vi "check asynchronous errors.vi"(8 "error in":errorcluster, 11 "Module Info In":T1) -> (0 "error out":errorcluster, 2 "safe state?":bool, 3 "Module Info Out":T1)   [LabVIEW 2013, in "Standard Engine Runtime.lvclass"]
uses:
  Standard Engine Runtime.lvclass
  async execution info.ctl
  asynchronous process data.ctl
  async command notification.ctl
  <vilib>/NI/Tag Bus/table/data table.ctl
  <vilib>/NI/Tag Bus Module Framework/runtime/execution settings.ctl
  async error info.ctl
  <vilib>/NI/Tag Bus Module Framework/runtime/error classification.ctl
  Data Table with Transfer Spec.ctl
  <vilib>/NI/Tag Bus/table/transfer specification.ctl
  <vilib>/NI/Tag Bus/tag/Data Type.ctl
  Configuration/Module Decimation.ctl
  Configuration/Module Error Configuration.ctl
  Configuration/Error Actions By Category.ctl
  Configuration/Error Actions.ctl
  Configuration/Standard Engine Configuration.lvclass
  <vilib>/NI/Tag Bus Module Framework/runtime/TBM module execution interface.lvclass
  <vilib>/NI/Tag Bus/tag/tag descriptor.lvclass
  <vilib>/NI/Tag Bus/table/data table.lvlib
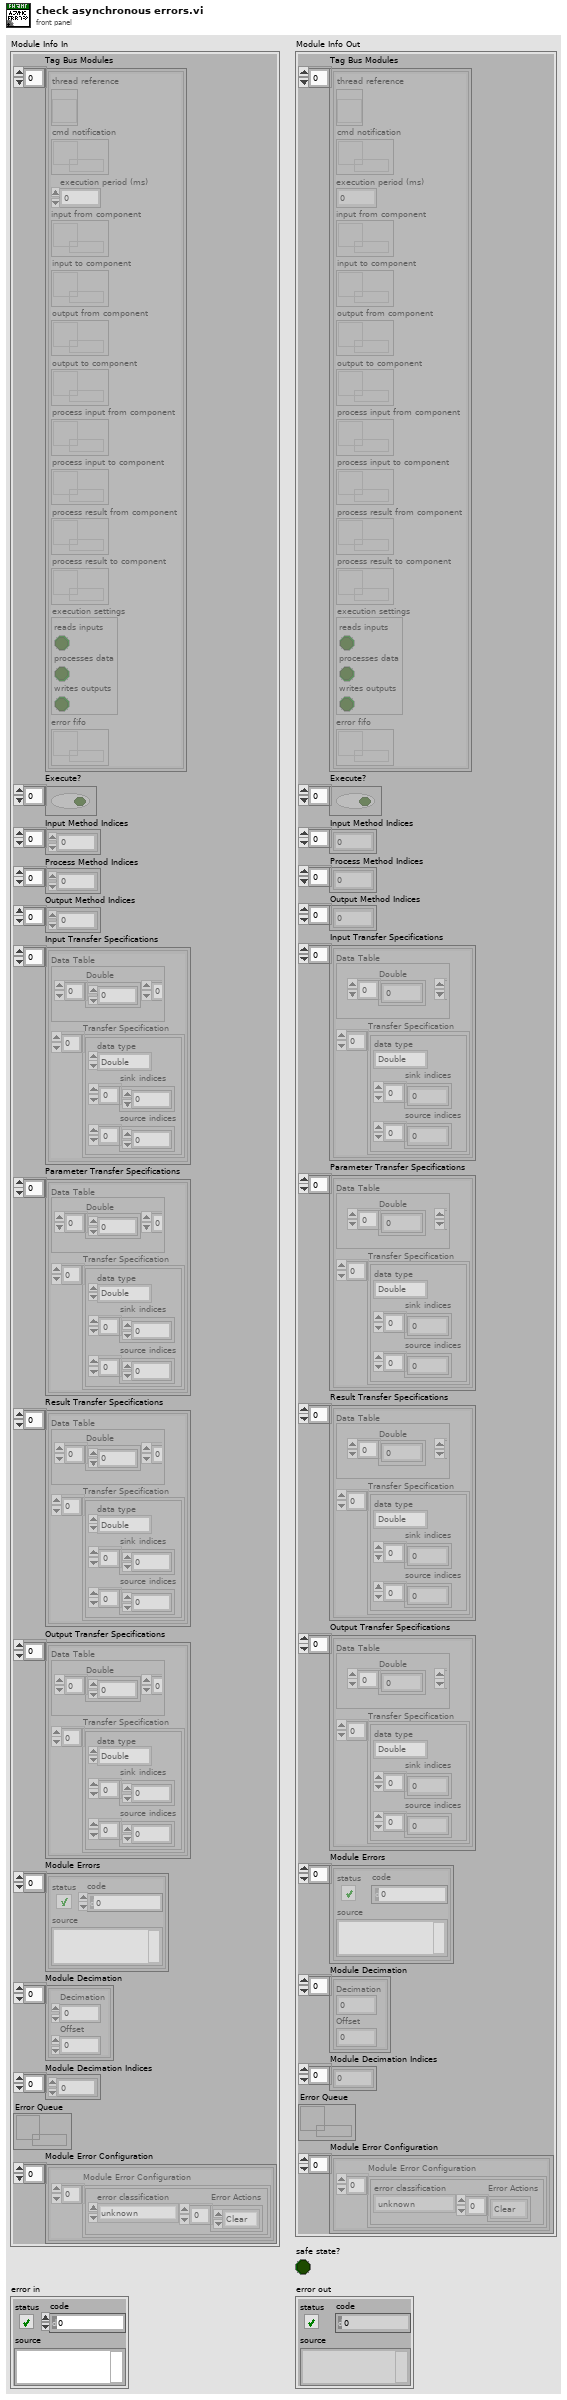
[diagram p1: front panel]
types:
  T1 = typedef "Standard Engine Runtime.lvclass/async execution info.ctl" = cluster{"Tag Bus Modules":T2[], "Execute?":bool[], "Input Method Indices":i32[], "Process Method Indices":i32[], "Output Method Indices":i32[], "Input Transfer Specifications":T4[], "Parameter Transfer Specifications":T4[], "Result Transfer Specifications":T4[], "Output Transfer Specifications":T4[], "Module Errors":errorcluster[], "Module Decimation":T8[], "Module Decimation Indices":i32[], "Error Queue":refnum<queue>, "Module Error Configuration":T9[]}
  T2 = typedef "Standard Engine Runtime.lvclass/asynchronous process data.ctl" = cluster{"thread reference":refnum<vi>, "cmd notification":refnum<k33>, "execution period (ms)":i32, "input from component":refnum<queue>, "input to component":refnum<queue>, "output from component":refnum<queue>, "output to component":refnum<queue>, "process input from component":refnum<queue>, "process input to component":refnum<queue>, "process result from component":refnum<queue>, "process result to component":refnum<queue>, "execution settings":T3, "error fifo":refnum<k33>}
  T3 = typedef "TBM module execution interface.lvclass/execution settings.ctl" = cluster{"reads inputs":bool, "processes data":bool, "writes outputs":bool}
  T4 = typedef "Standard Engine Runtime.lvclass/Data Table with Transfer Spec.ctl" = cluster{"Data Table":T5, "Transfer Specification":T6[]}
  T5 = typedef "tag bus.lvlib/data table.lvlib/data table.ctl" = cluster{"Double":dbl[], "Single":sgl[], "I64":i64[], "I32":i32[], "I16":i16[], "I8":i8[], "U64":u64[], "U32":u32[], "U16":u16[], "U8":u8[], "Boolean":bool[], "String":string[], "Array of Double":cluster{"DBL Array":dbl[]}[], "Array of Single":cluster{"SGL Array":sgl[]}[], "Array of I64":cluster{"I64 Array":i64[]}[], "Array of I32":cluster{"I32 Array":i32[]}[], "Array of I16":cluster{"I16 Array":i16[]}[], "Array of I8":cluster{"I8 Array":i8[]}[], "Array of U64":cluster{"U64 Array":u64[]}[], "Array of U32":cluster{"U32 Array":u32[]}[], "Array of U16":cluster{"U16 Array":u16[]}[], "Array of U8":cluster{"U8 Array":u8[]}[], "Array of Boolean":cluster{"Boolean Array":bool[]}[], "Array of String":cluster{"String Array":string[]}[]}
  T6 = typedef "tag bus.lvlib/data table.lvlib/transfer specification.ctl" = cluster{"data type":T7, "sink indices":i32[], "source indices":i32[]}
  T7 = typedef "tag bus.lvlib/tag descriptor.lvclass/Data Type.ctl" = enum16{"Double", "Single", "I64", "I32", "I16", "I8", "U64", "U32", "U16", "U8", "Boolean", "String", "Array of Double", "Array of Single", "Array of I64", "Array of I32", "Array of I16", "Array of I8", "Array of U64", "Array of U32", "Array of U16", "Array of U8", "Array of Boolean", "Array of String"}
  T8 = typedef "Standard Engine Configuration.lvclass/Module Decimation.ctl" = cluster{"Decimation":u16, "Offset":u16}
  T9 = typedef "Standard Engine Configuration.lvclass/Module Error Configuration.ctl" = cluster{"Module Error Configuration":T10[]}
  T10 = typedef "Standard Engine Configuration.lvclass/Error Actions By Category.ctl" = cluster{"error classification":T11, "Error Actions":T12[]}
  T11 = typedef "TBM module execution interface.lvclass/error classification.ctl" = enum16{"unknown", "none", "trivial", "recoverable", "critical"}
  T12 = typedef "Standard Engine Configuration.lvclass/Error Actions.ctl" = enum16{"Clear", "Notify", "Stop Component", "Stop Engine", "Safe State", "Attempt Recovery"}
  T13 = typedef "Standard Engine Runtime.lvclass/async error info.ctl" = cluster{"error code":i32, "error classification":T11}
  T14 = typedef "Standard Engine Runtime.lvclass/async command notification.ctl" = enum16{"stop", "safe state", "recover", "clear error"}
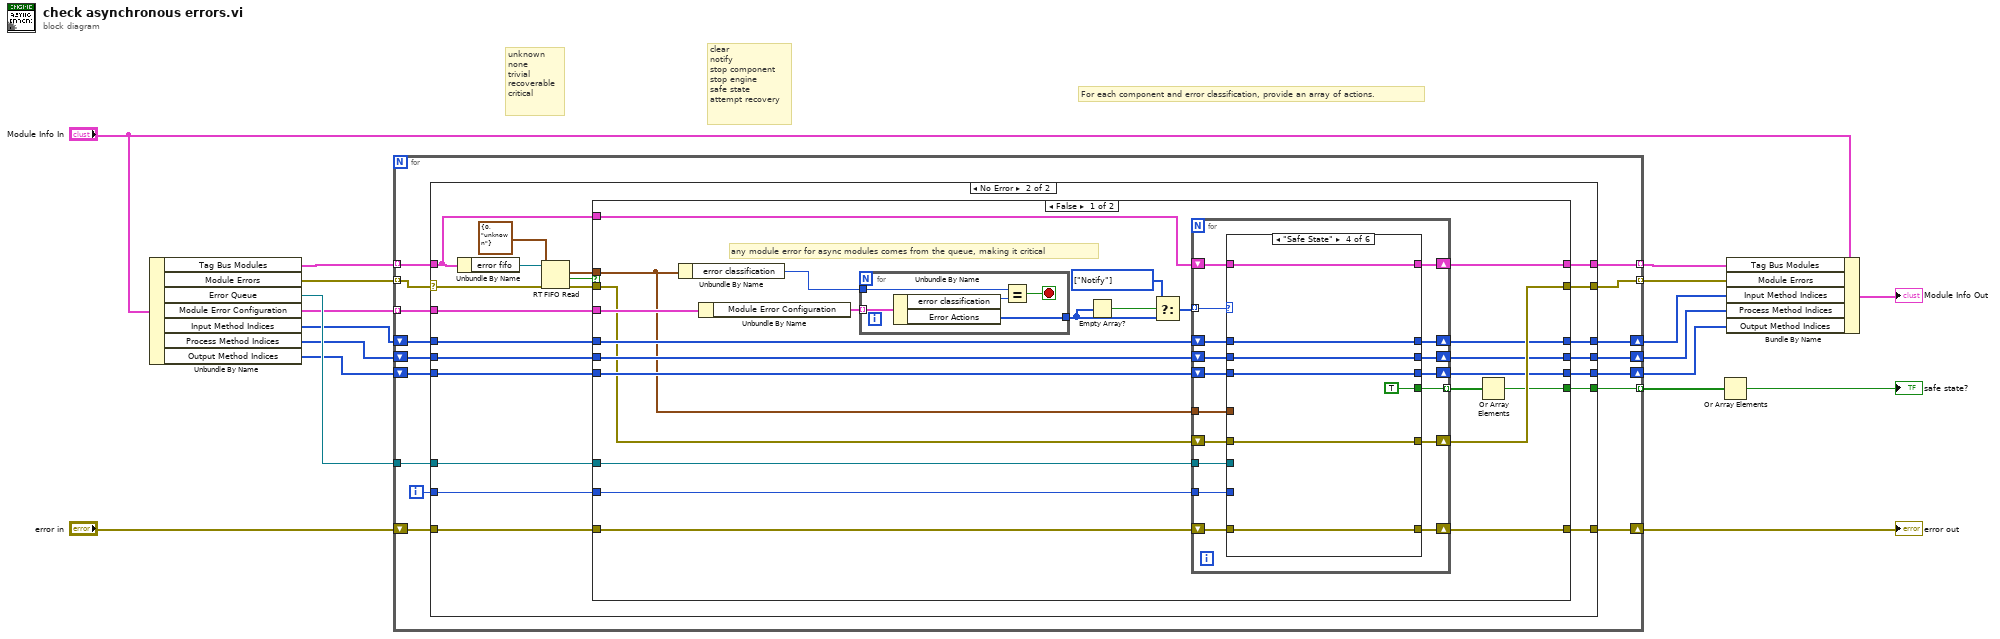
[diagram p0: block diagram]
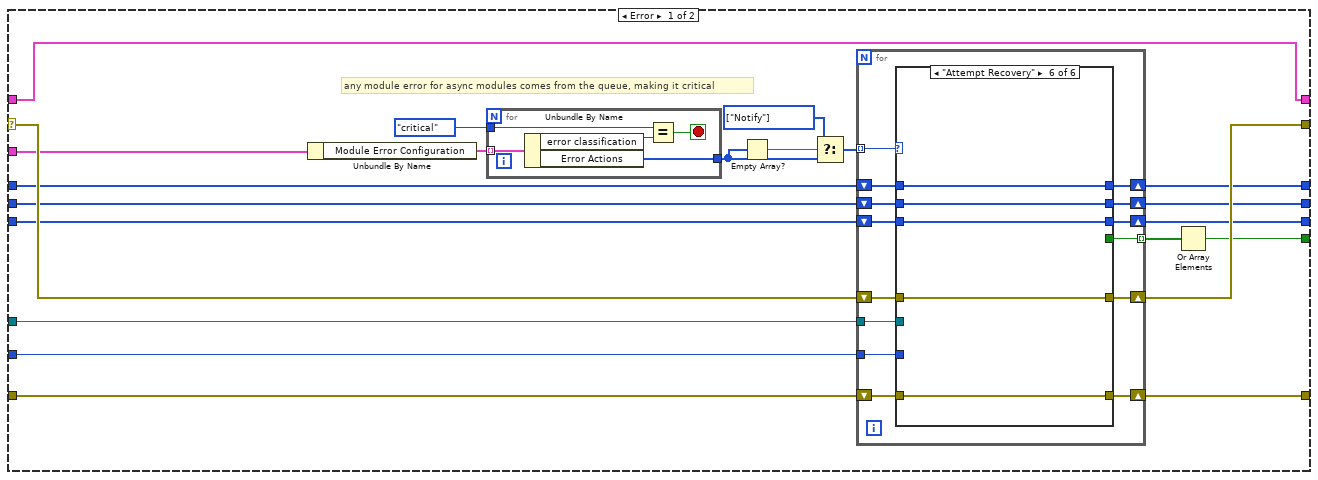
[diagram p2: hidden frame]
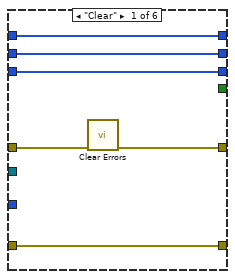
[diagram p3: hidden frame]
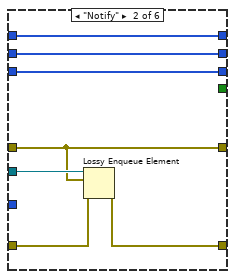
[diagram p4: hidden frame]
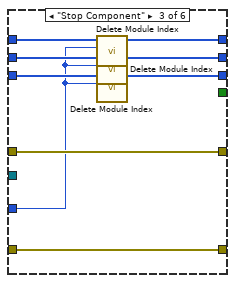
[diagram p5: hidden frame]
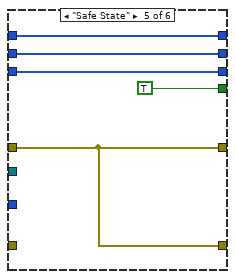
[diagram p7: hidden frame]
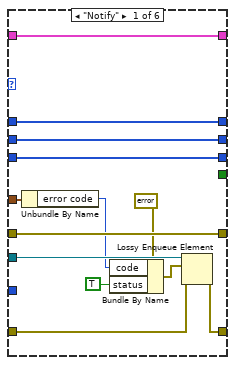
[diagram p8: hidden frame]
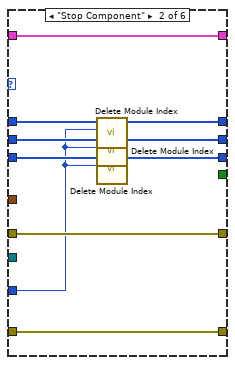
[diagram p9: hidden frame]
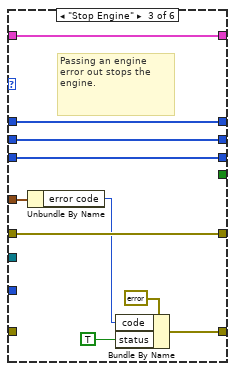
[diagram p10: hidden frame]
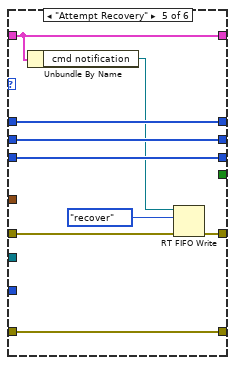
[diagram p11: hidden frame]
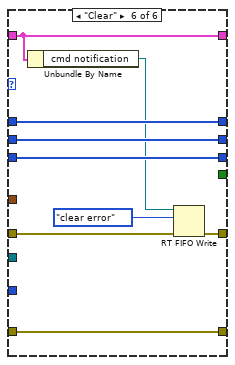
[diagram p12: hidden frame]
diagram:
  # "clear\nnotify\nstop component\nstop engine\nsafe state\nattempt recovery"
  # "unknown\nnone\ntrivial\nrecoverable\ncritical"
  # "For each component and error classification, provide an array of actions."
  n1 = Unbundle By Name("Module Info In") -> ("Tag Bus Modules"=w17:T2[], "Module Errors"=w16:errorcluster[], "Error Queue"=w15:refnum<queue>, "Module Error Configuration"=w12:T9[], "Input Method Indices"=w11:i32[], "Process Method Indices"=w10:i32[], "Output Method Indices"=w9:i32[])
  n2 = for {
    tunnel: w16 -> [w27] mode=indexing
    tunnel: [w32] -> w13 mode=indexing
    tunnel: [w31] -> w14 mode=indexing
    tunnel: w17 -> [w29] mode=indexing
    tunnel: w12 -> [w30] mode=indexing
    tunnel: [w28] -> w18 mode=indexing
    shift-right: [w33] -> w3
    shift-left: "error in" -> [w34]
    tunnel: w15 -> [w26]
    shift-right: [w22] -> w8
    shift-left: w11 -> [w25]
    shift-right: [w21] -> w7
    shift-left: w10 -> [w24]
    shift-right: [w20] -> w6
    shift-left: w9 -> [w23]
    i -> [w19]
    n3 = case shown="No Error" w27 {
      selector: w27 -> [w51 w128]
      tunnel: w34 -> [w53 w130]
      tunnel: [w52 w129] -> w33
      tunnel: [w56 w132] -> w32
      tunnel: [w36 w112] -> w31
      tunnel: w29 -> [w36 w113]
      tunnel: w30 -> [w42 w119]
      tunnel: [w55 w131] -> w28
      tunnel: w26 -> [w50 w127]
      tunnel: w25 -> [w49 w126]
      tunnel: w24 -> [w48 w125]
      tunnel: w23 -> [w47 w124]
      tunnel: [w46 w123] -> w22
      tunnel: [w45 w122] -> w21
      tunnel: [w44 w121] -> w20
      tunnel: w19 -> [w43 w120]
      frame Error {
        w37 = T12[] [enum."Notify"] items=["Clear", "Notify", "Stop Component", "Stop Engine", "Safe State", "Attempt Recovery"] ("t")
        # "any module error for async modules comes from the queue, making it critical"
        n4 = Unbundle By Name(w42) -> ("Module Error Configuration"=w41:T10[])
        n5 = for {
          tunnel: w41 -> [w61] mode=indexing
          tunnel: error_classification."critical" ("error classification") -> [w60]
          tunnel: [w57] -> w39
          stop <- w58 stop-if-true
          n6 = Unbundle By Name(w61) -> ("error classification"=w59:T11, "Error Actions"=w57:T12[])
          n7 = Equal?(x=w60, y=w59) -> (x = y?=w58:bool)
        }
        n8 = Empty Array?(array=w39) -> (empty?=w40:bool)
        n9 = Select(t=w37, s=w40, f=w39) -> (s? t:f=w38:T12[])
        n10 = for {
          tunnel: w38 -> [w75] mode=indexing
          tunnel: [w72] -> w54 mode=indexing
          shift-right: [w74] -> w56
          shift-left: w51 -> [w73]
          shift-right: [w70] -> w52
          shift-left: w53 -> [w71]
          tunnel: w50 -> [w69]
          shift-right: [w67] -> w46
          shift-left: w49 -> [w68]
          shift-right: [w65] -> w45
          shift-left: w48 -> [w66]
          shift-right: [w63] -> w44
          shift-left: w47 -> [w64]
          tunnel: w43 -> [w62]
          n11 = case shown="\"Attempt Recovery\"" w75 {
            tunnel: [w80 w82 w97 w101 w105 w111] -> w74
            tunnel: w73 -> [w81 w82 w97 w101 w105 w111]
            tunnel: [_ _ _ _ TRUE ("Stop Engine") _] -> w72
            tunnel: w71 -> [w79 w83 w96 _ _ w110]
            tunnel: [w79 w87 w96 w101 w105 w110] -> w70
            tunnel: w69 -> [_ w88 _ _ _ _]
            tunnel: w68 -> [w78 w86 w95 w100 w104 w109]
            tunnel: [w78 w86 w94 w100 w104 w109] -> w67
            tunnel: w66 -> [w77 w85 w93 w99 w103 w108]
            tunnel: [w77 w85 w91 w99 w103 w108] -> w65
            tunnel: w64 -> [w76 w84 w92 w98 w102 w107]
            tunnel: [w76 w84 w90 w98 w102 w107] -> w63
            tunnel: w62 -> [_ _ w89 _ _ _]
            frame "Clear" {
              n12 = call <vilib>:"Clear Errors.vi"("error in (no error)"=w81) -> ("error out"=w80:errorcluster)  [unwired: 6 in]
            }
            frame "Notify" {
              n13 = Lossy Enqueue Element(queue=w88, element=w82, error in (no error)=w83) -> (error out=w87:errorcluster)  [unwired: 3 out]
            }
            frame "Stop Component" {
              n14 = call "Delete Module Index.vi"("Index"=w89, "Module Indices"=w95) -> ("Module Indices"=w94:i32[])  [unwired: 9 in]
              n15 = call "Delete Module Index.vi"("Index"=w89, "Module Indices"=w93) -> ("Module Indices"=w91:i32[])  [unwired: 9 in]
              n16 = call "Delete Module Index.vi"("Index"=w89, "Module Indices"=w92) -> ("Module Indices"=w90:i32[])  [unwired: 9 in]
            }
            frame "Stop Engine" {
              # "Passing an engine error out stops the engine."
            }
            frame "Safe State" {
            }
            frame "Attempt Recovery" {
            }
          }
        }
        n17 = Or Array Elements(Boolean array=w54) -> (logical OR=w55:bool)
      }
      frame No Error {
        n18 = Unbundle By Name(w113) -> ("error fifo"=w117:refnum<k33>)
        n19 = RT FIFO Read(0:w117, 1:T13 {"error code"=0, "error classification"=enum."unknown"} ("element"), 3:w128) -> (9:w114:T13, 10:w115:bool, 11:w118:errorcluster)  [unwired: 1 in, 2 out]
        n20 = case shown="False" w115 {
          tunnel: [w156 w241] -> w132
          tunnel: [w155 _] -> w131
          tunnel: w130 -> [w153 w237]
          tunnel: [w152 w237] -> w129
          tunnel: w127 -> [w151 _]
          tunnel: w126 -> [w150 w240]
          tunnel: w125 -> [w149 w239]
          tunnel: w124 -> [w148 w238]
          tunnel: [w147 w240] -> w123
          tunnel: [w146 w239] -> w122
          tunnel: [w145 w238] -> w121
          tunnel: w120 -> [w144 _]
          tunnel: w119 -> [w143 _]
          tunnel: w118 -> [w137 w241]
          tunnel: w114 -> [w133 _]
          tunnel: w113 -> [w136 w242]
          tunnel: [w135 w242] -> w112
          frame False {
            w138 = T12[] [enum."Notify"] items=["Clear", "Notify", "Stop Component", "Stop Engine", "Safe State", "Attempt Recovery"] ("t")
            # "any module error for async modules comes from the queue, making it critical"
            n21 = Unbundle By Name(w133) -> ("error classification"=w134:T11)
            n22 = Unbundle By Name(w143) -> ("Module Error Configuration"=w142:T10[])
            n23 = for {
              tunnel: w142 -> [w161] mode=indexing
              tunnel: w134 -> [w160]
              tunnel: [w157] -> w140
              stop <- w158 stop-if-true
              n24 = Unbundle By Name(w161) -> ("error classification"=w159:T11, "Error Actions"=w157:T12[])
              n25 = Equal?(x=w160, y=w159) -> (x = y?=w158:bool)
            }
            n26 = Empty Array?(array=w140) -> (empty?=w141:bool)
            n27 = Select(t=w138, s=w141, f=w140) -> (s? t:f=w139:T12[])
            n28 = for {
              tunnel: w139 -> [w178] mode=indexing
              tunnel: [w175] -> w154 mode=indexing
              shift-right: [w177] -> w156
              shift-left: w137 -> [w176]
              shift-right: [w173] -> w152
              shift-left: w153 -> [w174]
              tunnel: w151 -> [w172]
              shift-right: [w170] -> w147
              shift-left: w150 -> [w171]
              shift-right: [w168] -> w146
              shift-left: w149 -> [w169]
              shift-right: [w166] -> w145
              shift-left: w148 -> [w167]
              tunnel: w144 -> [w165]
              shift-right: [w162] -> w135
              shift-left: w136 -> [w163]
              tunnel: w133 -> [w164]
              n29 = case shown="\"Safe State\"" w178 {
                tunnel: [w185 w201 w211 w217 w221 w230] -> w177
                tunnel: w176 -> [w185 w201 w211 w217 w227 w236]
                tunnel: [_ _ _ TRUE ("Stop Engine") _ _] -> w175
                tunnel: w174 -> [w186 w200 _ w212 w226 w235]
                tunnel: [w190 w200 w202 w212 w226 w235] -> w173
                tunnel: w172 -> [w191 _ _ _ _ _]
                tunnel: w171 -> [w189 w199 w210 w216 w225 w234]
                tunnel: [w189 w198 w210 w216 w225 w234] -> w170
                tunnel: w169 -> [w188 w197 w209 w215 w224 w233]
                tunnel: [w188 w195 w209 w215 w224 w233] -> w168
                tunnel: w167 -> [w187 w196 w208 w214 w223 w232]
                tunnel: [w187 w194 w208 w214 w223 w232] -> w166
                tunnel: w165 -> [_ w193 _ _ _ _]
                tunnel: w164 -> [w180 _ w203 _ _ _]
                tunnel: w163 -> [w184 w192 w207 w213 w222 w231]
                tunnel: [w184 w192 w207 w213 w222 w231] -> w162
                frame "Notify" {
                  n30 = Unbundle By Name(w180) -> ("error code"=w179:i32)
                  n31 = Bundle By Name(cluster=errorcluster {"status"=FALSE, "code"=0, "source"=""} ("element"), "code"=w179, "status"=TRUE) -> (w182:errorcluster)
                  n32 = Lossy Enqueue Element(queue=w191, element=w182, error in (no error)=w186) -> (error out=w190:errorcluster)  [unwired: 3 out]
                }
                frame "Stop Component" {
                  n33 = call "Delete Module Index.vi"("Index"=w193, "Module Indices"=w199) -> ("Module Indices"=w198:i32[])  [unwired: 9 in]
                  n34 = call "Delete Module Index.vi"("Index"=w193, "Module Indices"=w197) -> ("Module Indices"=w195:i32[])  [unwired: 9 in]
                  n35 = call "Delete Module Index.vi"("Index"=w193, "Module Indices"=w196) -> ("Module Indices"=w194:i32[])  [unwired: 9 in]
                }
                frame "Stop Engine" {
                  # "Passing an engine error out stops the engine."
                  n36 = Unbundle By Name(w203) -> ("error code"=w204:i32)
                  n37 = Bundle By Name(cluster=errorcluster {"status"=FALSE, "code"=0, "source"=""} ("element"), "code"=w204, "status"=TRUE) -> (w202:errorcluster)
                }
                frame "Safe State" {
                }
                frame "Attempt Recovery" {
                  n38 = Unbundle By Name(w222) -> ("cmd notification"=w220:refnum<k33>)
                  n39 = RT FIFO Write(0:w220, 1:async_command_notification."recover" ("notification"), 3:w227) -> (11:w221:errorcluster)  [unwired: 2 in, 3 out]
                }
                frame "Clear" {
                  n40 = Unbundle By Name(w231) -> ("cmd notification"=w229:refnum<k33>)
                  n41 = RT FIFO Write(0:w229, 1:async_command_notification."clear error" ("notification"), 3:w236) -> (11:w230:errorcluster)  [unwired: 2 in, 3 out]
                }
              }
            }
            n42 = Or Array Elements(Boolean array=w154) -> (logical OR=w155:bool)
          }
          frame True {
          }
        }
      }
    }
  }
  "error out" <- w3
  n43 = Or Array Elements(Boolean array=w18) -> (logical OR=→"safe state?":bool)
  n44 = Bundle By Name(cluster="Module Info In", "Tag Bus Modules"=w14, "Module Errors"=w13, "Input Method Indices"=w8, "Process Method Indices"=w7, "Output Method Indices"=w6) -> (→"Module Info Out":T1)
